vi "PID_2_Channels_Sequence_New.vi"() -> ()   [LabVIEW 2016]
uses:
  <vilib>/Analysis/3filter.llb/Filter Passband Type.ctl
  <vilib>/Analysis/baseanly.llb/Mean (DBL).vi
  <vilib>/addons/control/pid/pid.llb/PID Advanced (DBL Array).vi
  <vilib>/addons/control/pid/pid.llb/PID Parameter Manager (DBL Array).vi
  <vilib>/addons/control/pid/pid.llb/PID Derivative Action Buffered (DBL Array).vi
  <vilib>/addons/control/pid/pid.llb/PID Get Advanced Error (DBL Array).vi
  <vilib>/addons/control/pid/pid.llb/PID Integral Action Buffered (DBL Array).vi
  <vilib>/addons/control/pid/pid.llb/PID Resize 1D Array.vi
  <vilib>/addons/control/pid/pid.llb/PID Get Advanced Error (DBL).vi
  <userlib>/Fluigent/Fluigent MFCS/FluigentMFCS_Full.llb/MFCS_EZ Detect.vi
  <userlib>/Fluigent/Fluigent MFCS/FluigentMFCS_Full.llb/MFCS_EZ Initialization.vi
  <userlib>/Fluigent/Fluigent MFCS/FluigentMFCS_Full.llb/MFCS_EZ Write Channel Pressure.vi
  PID2ChanGlobals.vi
  <userlib>/Fluigent/Fluigent MFCS/FluigentMFCS_Full.llb/MFCS_EZ Read Channel Pressure.vi
  <vilib>/Analysis/3filter.llb/Butterworth Filter (DBL).vi
  <vilib>/Analysis/NI_AALBase.lvlib
  <vilib>/addons/control/pid/NI_PID_pid.lvlib
panel:
  in  "output range":cluster{"output high":dbl, "output low":dbl}[](array[cluster])=[{"output high"=100.0, "output low"=-100.0}] {"output low" format="%.2f"; "output high" format="%.2f"}
  out "Err Signal":dbl[][](graph)
  in  "Control Pressure Set":dbl=235.0
  in  "Set current pressures to manual pressure":bool
  out "dP/dt":dbl[](graph)
  in  "Fwater (measured)":dbl=600.0
  out "Ratio":dbl[](graph)
  out "F0":dbl[](graph)
  out "Flow Setpoints":dbl[](array[numeric])=[200.784, 133.856]
  in  "Manual Total Mix Flow":dbl=300.0
  out "Total Set Mix Flow":dbl=334.64
  in  "Add Ctrl?":bool=TRUE
  in  "setpoint range":T1(array[cluster])=[{"setpoint high"=1200.0, "setpoint low"=0.0}, {"setpoint high"=1200.0, "setpoint low"=0.0}] {"setpoint high" format="%.2f"; "setpoint low" format="%.2f"}
  in  "Manual Pressure Set":dbl[](array[numeric])=[500.0, 500.0]
  in  "Pressure Channels":enum16{"1", "2", "3", "4"}[](array[ring])=[enum."1", enum."3"]
  in  "gamma":dbl[](array[numeric])=[0.0] format="%.2f"
  in  "linearity":dbl[](array[numeric])=[1.0] format="%.2f"
  in  "beta":dbl[](array[numeric])=[1.0] format="%.2f"
  in  "PID Gains":T2(array[cluster])=[{"Proportional Gain"=0.4, "Integral Time"=0.03, "Derivative Time"=0.0}, {"Proportional Gain"=0.4, "Integral Time"=0.03, "Derivative Time"=0.0}]
  in  "F0 set":dbl=900.0
  out "Current F2":dbl=128.94551724137932
  out "Current F0":dbl=832.3103448275862
  in  "Valves":enum16{"1", "2", "3", "4", "5", "6", "7", "8"}[](array[ring])=[enum."5", enum."4"]
  in  "Boards":enum16{"A", "B", "C"}[](array[ring])=[enum."A", enum."A"]
  out "error out":errorcluster
  out "dt":dbl=0.024001598358154297
  in  "Filter Size":i32=5
  out "Current F1":dbl=200.3448275862069
  in  "reinitialize? (F)":bool
  out "Flow Rates":dbl[][](graph)
  out "Pressure Setpoint":dbl[][](graph)
  in  "stop":bool
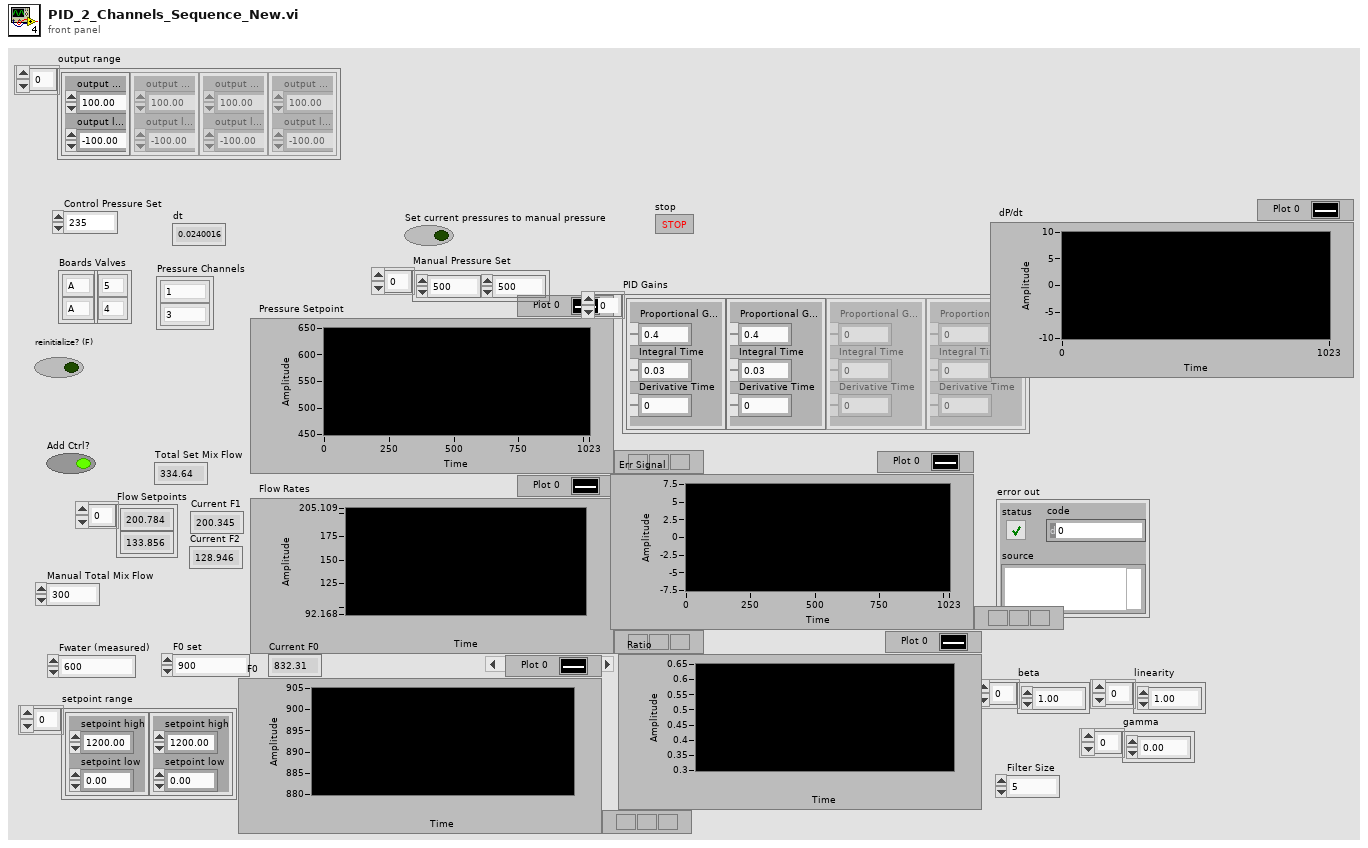
[diagram p1: front panel]
types:
  T1 = cluster{"setpoint high":dbl, "setpoint low":dbl}[]
  T2 = cluster{"Proportional Gain":dbl, "Integral Time":dbl, "Derivative Time":dbl}[]
  T3 = typedef "_EZmfcsSN.ctl" = u16
  T4 = typedef "_EZmfcsRefNum.ctl" = refnum<k1>
  T5 = typedef "_frpRefNum" = refnum<k1>
  T6 = typedef "NI_AALBase.lvlib/Filter Passband Type.ctl" = enum32{"Lowpass", "Highpass", "Bandpass", "Bandstop"}
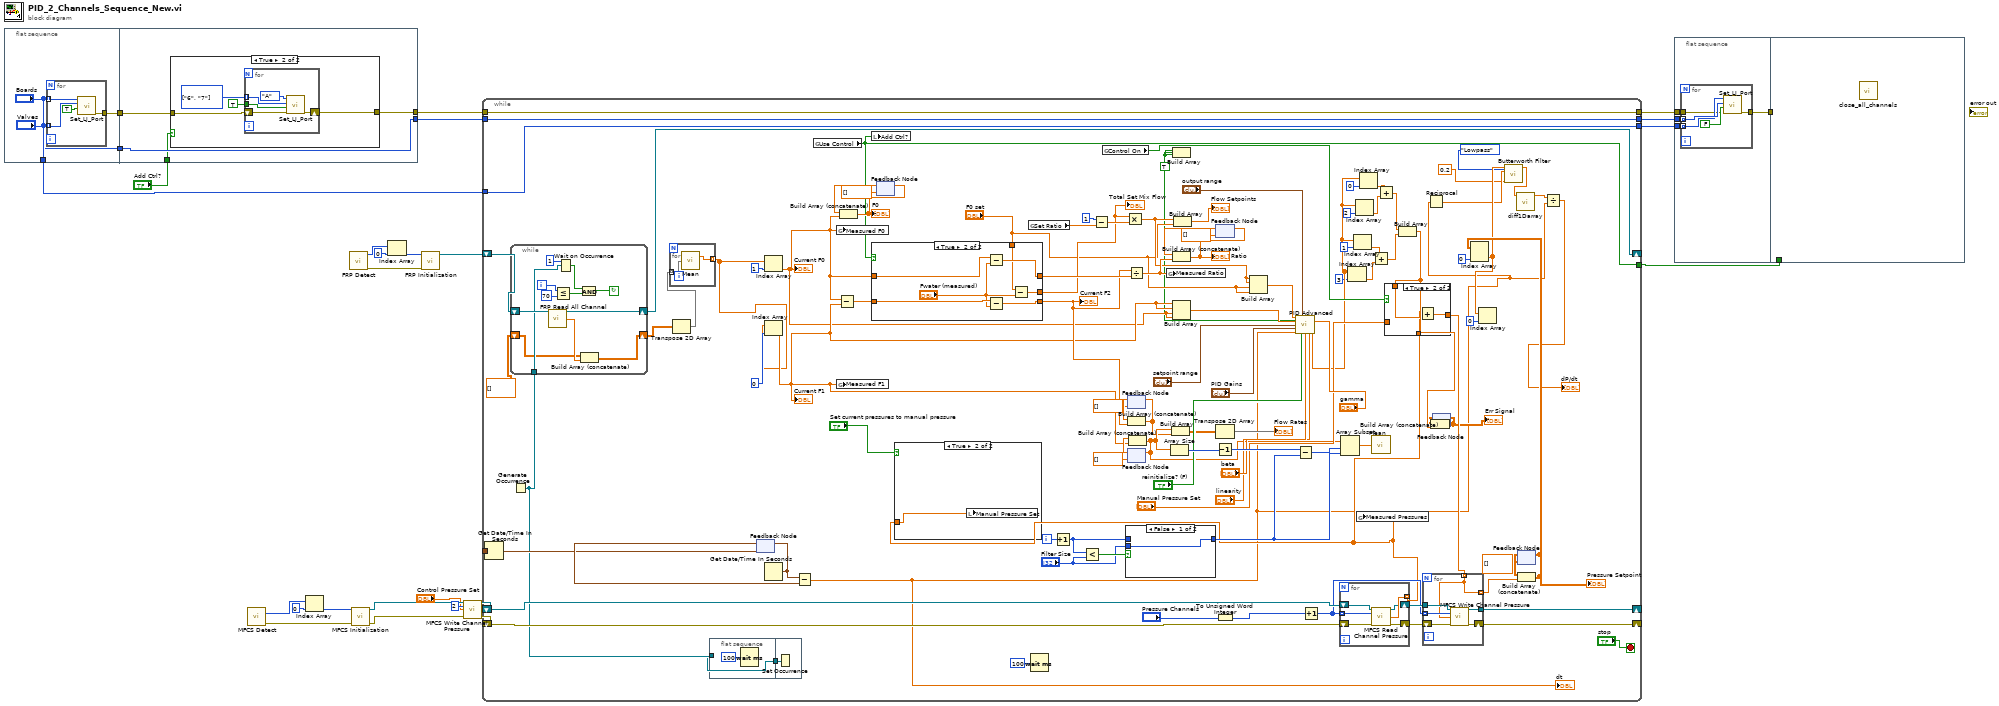
[diagram p0: block diagram]
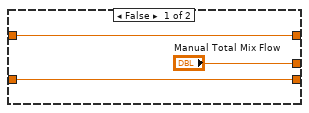
[diagram p4: hidden frame]
diagram:
  n1 = flat-sequence {
    tunnel: ["Boards"] -> w16
    tunnel: [w30] -> w11
    tunnel: ["Valves"] -> w10
    tunnel: [w38] -> w15
    tunnel: [w36] -> w17
    tunnel: w11 -> [w37]
    tunnel: w10 -> [w38]
    tunnel: "Add Ctrl?" -> [w35]
    frame #0 {
      n2 = for {
        tunnel: "Valves" -> [w34] mode=indexing
        tunnel: "Boards" -> [w33] mode=indexing
        tunnel: [w31] -> w30
        n3 = call "Set_LJ_Port.vi"("State"=TRUE, "Channel"=w34, "Flowboard"=w33) -> ("error out"=w31:errorcluster)  [unwired: 8 in]
      }
    }
    frame #1 {
      n4 = case shown="True" w35 {
        tunnel: w37 -> [w39 w43]
        tunnel: [w39 w42] -> w36
        frame False {
        }
        frame True {
          w40 = enum16{"1", "2", "3", "4", "5", "6", "7", "8"}[] [enum."6", enum."7"] items=["1", "2", "3", "4", "5", "6", "7", "8"]
          n5 = for {
            tunnel: TRUE ("State") -> [w46]
            shift-right: [w47] -> w42
            shift-left: w43 -> [w48]
            tunnel: w40 -> [w45] mode=indexing
            n6 = call "Set_LJ_Port.vi"("error in"=w48, "State"=w46, "Channel"=w45, "Flowboard"=enum16{"A", "B", "C"}."A") -> ("error out"=w47:errorcluster)  [unwired: 7 in]
          }
        }
      }
    }
  }
  n7 = call-poly <userlib>:"MFCS Detect.vi"() -> ("[SN MFCS_EZ]"=w27:T3[], "error out"=w25:errorcluster)  [unwired: 14 in]
  n8 = Index Array(array=w27, index=0) -> (element=w26:T3)
  n9 = call <userlib>:"FRP Detect.vi"() -> ("FLOWBOARD List"=w24:u16[], "error out"=w21:errorcluster)  [unwired: 14 in]
  n10 = call-poly <userlib>:"MFCS Initialization.vi"("SN MFCS_EZ"=w26, "error in (no error)"=w25) -> ("MFCS_EZ"=w6:T4, "error out"=w4:errorcluster)  [unwired: 11 in, 1 out]
  n11 = Index Array(array=w24, index=0) -> (element=w20:u16)
  n12 = call <userlib>:"FRP Initialization.vi"("Serial Number"=w20, "error in (no error)"=w21) -> ("FRP out"=w19:T5)  [unwired: 11 in, 2 out]
  n13 = call-poly <userlib>:"MFCS Write Channel Pressure.vi"("MFCS_EZ"=w6, "Channel Number (default=1)"=u8 2, "Pressure (mBar)"="Control Pressure Set", "error in (no error)"=w4) -> ("MFCS_EZ out"=w5:T4, "error out"=w3:errorcluster)  [unwired: 10 in]
  n14 = Get Date/Time In Seconds() -> (seconds since 1Jan1904=w18:timestamp)
  n15 = while {
    shift-right: [w132] -> _
    shift-left: w3 -> [w155]
    shift-right: [w130] -> _
    shift-left: w5 -> [w156]
    shift-right: [w152] -> _
    shift-left: w19 -> [w153]
    tunnel: [w136] -> w12
    tunnel: w17 -> [w136]
    tunnel: w18 -> [w122]
    tunnel: w16 -> [w137]
    tunnel: w15 -> [w138]
    tunnel: [w138] -> w14
    tunnel: [w137] -> w13
    tunnel: [w106] -> w7
    i -> [w147]
    stop <- "stop" stop-if-true
    w58 = TRUE ("Control On")
    n16 = Generate Occurrence() -> (w54:refnum<k4>)
    n17 = while {
      shift-right: [w169] -> w152
      shift-left: w153 -> [w170]
      tunnel: w54 -> [w167]
      shift-right: [w159] -> w50
      shift-left: dbl[][] [] -> [w160]
      i -> [w161]
      stop <- w163 continue-if-true
      n18 = call <userlib>:"FRP Read All Channel.vi"("FRP"=w170) -> ("FRP out"=w169:T5, "All Flow-Rates"=w168:dbl[])  [unwired: 12 in, 1 out]
      n19 = Less Or Equal?(x=w161, y=70 ("x")) -> (x <= y?=w164:bool)
      n20 = Wait on Occurrence(2:w167, 3:1 ("ms timeout (-1)")) -> (0:w165:bool)  [unwired: 1 in]
      n21 = And(x=w165, y=w164) -> (x .and. y?=w163:bool)
      n22 = Build Array (concatenate)(w160, w168) -> (w159:dbl[][])
    }
    n23 = Transpose 2D Array(2D array=w50) -> (transposed array=w49:dbl[][])
    n24 = for {
      tunnel: w49 -> [w158] mode=indexing
      tunnel: [w157] -> w55 mode=indexing
      n25 = call-poly <vilib>:"Mean.vi"("X"=w158) -> ("mean"=w157:dbl)  [unwired: 1 out]
    }
    n26 = flat-sequence {
      tunnel: w54 -> [w171]
      tunnel: [w171] -> w53
      tunnel: w53 -> [w173]
      frame #0 {
        n27 = Wait (ms)(milliseconds to wait=u32 100) -> ()  [unwired: 1 out]
      }
      frame #1 {
        n28 = Set Occurrence(w173) -> ()
      }
    }
    n29 = feedback #1(w122) -> (w148:timestamp)
    n30 = Get Date/Time In Seconds() -> (seconds since 1Jan1904=w149:timestamp)
    n31 = feedback-in #1(w149) -> ()
    n32 = Index Array(array=w55, index=1) -> (element=w80:dbl)
    "Current F0" <- w80
    n33 = Index Array(array=w55, index=0) -> (element=w81:dbl)
    "Current F1" <- w81
    n34 = Subtract(x=w149, y=w148) -> (x-y=w56:dbl)
    "dt" <- w56
    n35 = global read "PID2ChanGlobals.vi" "Use Control"() -> (w106:bool)
    n36 = global write "PID2ChanGlobals.vi" "Measured F0"(w80) -> ()
    n37 = global write "PID2ChanGlobals.vi" "Measured F1"(w81) -> ()
    n38 = Subtract(x=w80, y=w81) -> (x-y=w115:dbl)
    n39 = local write "Add Ctrl?"(w106) -> ()
    n40 = case shown="True" w106 {
      tunnel: w115 -> [w177 w184]
      tunnel: [w177 w183] -> w82
      tunnel: ["Manual Total Mix Flow" w180] -> w99
      tunnel: w80 -> [w175 w182]
      tunnel: [w175 w181] -> w110
      tunnel: "F0 set" -> [_ w178]
      frame False {
      }
      frame True {
        n41 = Subtract(x=w182, y="Fwater (measured)") -> (x-y=w181:dbl)
        n42 = Subtract(x=w184, y="Fwater (measured)") -> (x-y=w183:dbl)
        n43 = Subtract(x=w178, y="Fwater (measured)") -> (x-y=w180:dbl)
      }
    }
    "Current F2" <- w82
    "Total Set Mix Flow" <- w99
    n44 = feedback #2(dbl[] []) -> (w111:dbl[])
    n45 = Build Array (concatenate)(w111, w80) -> (w112:dbl[])
    "F0" <- w112
    n46 = feedback-in #2(w112) -> ()
    n47 = global read "PID2ChanGlobals.vi" "Set Ratio"() -> (w100:dbl)
    n48 = Wait (ms)(milliseconds to wait=u32 100) -> ()  [unwired: 1 out]
    n49 = Increment(x=w147) -> (x+1=w145:i32)
    n50 = Less?(x=w145, y="Filter Size") -> (x < y?=w146:bool)
    n51 = Subtract(x=1, y=w100) -> (x-y=w113:dbl)
    n52 = global read "PID2ChanGlobals.vi" "Control On"() -> (w105:bool)
    n53 = Multiply(x=w99, y=w113) -> (x*y=w79:dbl)
    n54 = case shown="False" w146 {
      tunnel: w145 -> [_ w202]
      tunnel: [w201 w202] -> w142
      tunnel: "Filter Size" -> [w201 _]
      frame False {
      }
      frame True {
      }
    }
    n55 = Divide(x=w82, y=w110) -> (x/y=w109:dbl)
    n56 = feedback #3(dbl[] []) -> (w121:dbl[])
    n57 = Build Array (concatenate)(w121, w82) -> (w103:dbl[])
    n58 = feedback-in #3(w103) -> ()
    n59 = feedback #4(dbl[] []) -> (w150:dbl[])
    n60 = Build Array (concatenate)(w150, w81) -> (w104:dbl[])
    n61 = feedback-in #4(w104) -> ()
    n62 = global write "PID2ChanGlobals.vi" "Measured Ratio"(w109) -> ()
    n63 = Array Size(array=w104) -> (size(s)=w143:i32)
    n64 = Build Array(w104, w103) -> (w102:dbl[][])
    n65 = Build Array(w58, w58) -> (w59:bool[])
    n66 = Build Array(w81, w81, w80, w80) -> (w116:dbl[])
    n67 = Build Array(w79, "F0 set") -> (→"Flow Setpoints":dbl[])
    n68 = feedback #5(dbl[] []) -> (w108:dbl[])
    n69 = Build Array (concatenate)(w108, w109) -> (w107:dbl[])
    "Ratio" <- w107
    n70 = feedback-in #5(w107) -> ()
    n71 = Transpose 2D Array(2D array=w102) -> (transposed array=→"Flow Rates":dbl[][])
    n72 = Decrement(x=w143) -> (x-1=w141:i32)
    n73 = To Unsigned Word Integer(number="Pressure Channels") -> (unsigned 16bit integer=w120:u16[])
    n74 = Build Array(w79, w79, "F0 set", "F0 set") -> (w76:dbl[])
    n75 = call-poly <vilib>:"PID Advanced.vi"("setpoint"=w76, "output range"="output range", "auto? (T)"=w59, "process variable"=w116, "gamma"="gamma", "setpoint range"="setpoint range", "PID gains"="PID Gains", "dt (s)"=w56, "reinitialize? (F)"="reinitialize? (F)", "beta"="beta", "linearity"="linearity") -> ("output"=w75:dbl[])  [unwired: 3 in, 1 out]
    n76 = Subtract(x=w141, y=w142) -> (x-y=w140:i32)
    n77 = Increment(x=w120) -> (x+1=w123:u16[])
    n78 = for {
      tunnel: [w192] -> w64 mode=indexing
      shift-right: [w191] -> w134
      shift-left: w156 -> [w194]
      shift-right: [w190] -> w133
      shift-left: w155 -> [w193]
      tunnel: w123 -> [w189] mode=indexing
      n79 = call-poly <userlib>:"MFCS Read Channel Pressure.vi"("MFCS_EZ"=w194, "Channel Number (default=1)"=w189, "error in (no error)"=w193) -> ("MFCS_EZ out"=w191:T4, "Pressure (mBar)"=w192:dbl, "error out"=w190:errorcluster)  [unwired: 9 in, 1 out]
    }
    n80 = case shown="True" "Set current pressures to manual pressure" {
      tunnel: w64 -> [_ w174]
      frame False {
      }
      frame True {
        n81 = local write "Manual Pressure Set"(w174) -> ()
      }
    }
    n82 = Array Subset(array=w104, index=w140, length=w142) -> (w139:dbl[])
    n83 = Index Array(array=w75, index=3) -> (element=w67:dbl)
    n84 = Index Array(array=w75, index=1) -> (element=w68:dbl)
    n85 = Index Array(array=w75, index=2) -> (element=w69:dbl)
    n86 = global write "PID2ChanGlobals.vi" "Measured Pressures"(w64) -> ()
    n87 = Index Array(array=w75, index=0) -> (element=w70:dbl)
    n88 = call-poly <vilib>:"Mean.vi"("X"=w139) -> ()  [unwired: 2 out]
    n89 = Add(x=w68, y=w67) -> (x+y=w65:dbl)
    n90 = Add(x=w70, y=w69) -> (x+y=w66:dbl)
    n91 = Build Array(w66, w65) -> (w62:dbl[])
    n92 = case shown="True" w105 {
      tunnel: "Manual Pressure Set" -> [w185 _]
      tunnel: [w185 w186] -> w118
      tunnel: w62 -> [_ w188]
      tunnel: w64 -> [_ w187]
      frame False {
      }
      frame True {
        n93 = Add(x=w187, y=w188) -> (x+y=w186:dbl[])
      }
    }
    n94 = for {
      tunnel: w134 -> [w200]
      shift-right: [w198] -> w132
      shift-left: w133 -> [w199]
      tunnel: [w195] -> w63 mode=indexing
      tunnel: [w197] -> w130
      tunnel: w123 -> [w196] mode=indexing
      tunnel: w118 -> [w195] mode=indexing
      n95 = call-poly <userlib>:"MFCS Write Channel Pressure.vi"("MFCS_EZ"=w200, "Channel Number (default=1)"=w196, "Pressure (mBar)"=w195, "error in (no error)"=w199) -> ("MFCS_EZ out"=w197:T4, "error out"=w198:errorcluster)  [unwired: 10 in]
    }
    n96 = Reciprocal(x=w56) -> (1/x=w92:dbl)
    n97 = feedback #6() -> (w61:dbl[][])  [unwired: 1 in]
    n98 = Build Array (concatenate)(w61, w62) -> (w60:dbl[][])
    "Err Signal" <- w60
    n99 = feedback-in #6(w60) -> ()
    n100 = feedback #7(dbl[][] []) -> (w131:dbl[][])
    n101 = Build Array (concatenate)(w131, w63) -> (w98:dbl[][])
    "Pressure Setpoint" <- w98
    n102 = Index Array(array=w98, index (col)=0 ("disabled index (col)")) -> (element=w93:dbl[])  [unwired: 1 in]
    n103 = Index Array(array=w93, index=0) -> ()  [unwired: 1 out]
    n104 = call-poly <vilib>:"Butterworth Filter.vi"("filter type"=Filter_Passband_Type."Lowpass", "low cutoff freq: fl"=0.2 ("high cutoff freq: fh"), "sampling freq: fs"=w92, "X"=w93) -> ("Filtered X"=w89:dbl[])  [unwired: 4 in, 1 out]
    n105 = call "diff1Darray.vi"("Input"=w89) -> ("Diff"=w95:dbl[])  [unwired: 10 in]
    n106 = feedback-in #7(w98) -> ()
    n107 = Divide(x=w95, y=w56) -> (x/y=→"dP/dt":dbl[])
  }
  n108 = flat-sequence {
    tunnel: w14 -> [w206]
    tunnel: w13 -> [w205]
    tunnel: w12 -> [w204]
    tunnel: [w203] -> w8
    tunnel: w8 -> [_]
    tunnel: w7 -> [_]
    frame #0 {
      n109 = for {
        tunnel: w206 -> [w211] mode=indexing
        tunnel: [w209] -> w203
        tunnel: w205 -> [w208] mode=indexing
        tunnel: w204 -> [w207]
        n110 = call "Set_LJ_Port.vi"("error in"=w207, "State"=FALSE, "Channel"=w211, "Flowboard"=w208) -> ("error out"=w209:errorcluster)  [unwired: 7 in]
      }
    }
    frame #1 {
      n111 = call "close_all_channels.vi"() -> ()  [unwired: 12 in]
    }
  }
